vi "Client Close.vi"(8 "error in":errorcluster, 11 "connection ID":T1) -> (0 "error out":errorcluster)   [LabVIEW 2010, in "NI_CCC.lvlib"]
doc: "Closes the connection with the server."
uses:
  NI_CCC.lvlib
  Connection ID.ctl
  <vilib>/NI/STM/TCP/TCP Connection Info.ctl
  <vilib>/NI/STM/SubVIs/MetaDataElement.ctl
  Tag Configuration.ctl
  <vilib>/NI/Current Value Table/Type Defs/Data Types.ctl
  Tag Direction.ctl
  FG Client Configurations Action.ctl
  <vilib>/NI/STM/TCP/TCP Write Options.ctl
  <vilib>/NI/Current Value Table/FGVs/Group Memory.vi
  <vilib>/NI/STM/NI STM.lvlib
  <vilib>/NI/Current Value Table/Current Value Table.lvlib
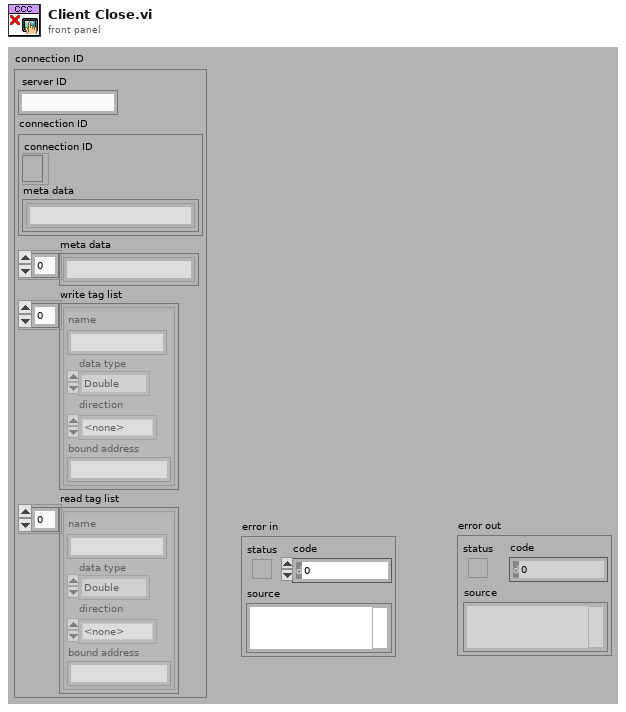
[diagram p1: front panel]
types:
  T1 = typedef "NI_CCC.lvlib/Connection ID.ctl" = cluster{"server ID":string, "connection ID":T2, "meta data":T3[], "write tag list":T4[], "read tag list":T4[]}
  T2 = typedef "NI STM.lvlib/TCP Connection Info.ctl" = cluster{"connection ID":refnum<k5>, "meta data":T3[]}
  T3 = typedef "NI STM.lvlib/MetaDataElement.ctl" = string
  T4 = typedef "NI_CCC.lvlib/Tag Configuration.ctl" = cluster{"name":string, "data type":T5, "direction":T6, "bound address":string}
  T5 = typedef "Current Value Table.lvlib/Data Types.ctl" = enum16{"Double", "Single", "I64", "I32", "I16", "I8", "U64", "U32", "U16", "U8", "String", "Boolean", "Array of U8", "Array of U16", "Array of U32", "Array of U64", "Array of I64", "Array of I32", "Array of I16", "Array of I8", "Array of Double", "Array of Single", "Array of Boolean", "Array of String"}
  T6 = typedef "NI_CCC.lvlib/Tag Direction.ctl" = enum32{"<none>", "Read", "Write"}
  T7 = typedef "NI_CCC.lvlib/FG Client Configurations Action.ctl" = enum16{"Check Read Config", "Check Write Config", "Mark Read Config", "Mark Write Config"}
  T8 = typedef "NI STM.lvlib/TCP Write Options.ctl" = cluster{"ignore timeout error":bool, "timeout ms (1000)":i32}
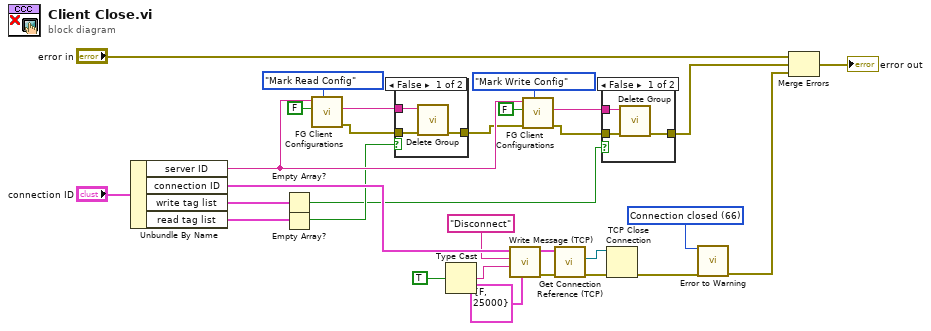
[diagram p0: block diagram]
diagram:
  w27 = 66 items=["No Error", "Argument Error", "Memory Full", "Out of Zone", "End of File", "File Already Open", "Generic File IO Error", "File Not Found", "File Permission Error", "Disk Full", "Duplicate Path", "Too Many Files Open", "Not Enabled", "Resource File Not Found", "Cannot Add Resource", "Resource Not Found", "Image Not Found", "Image Memory Error", "Pen Does Not Exist", "Config Bad Type", "Config Token Not Found", "Config Parse Error", "Config Memory Error", "Bad External Code Format", "Bad External Code Offset", "External Code Not Present", "Null Window", "Destroy Window Mixup", "Null Menu", "Print Aborted", "Bad Print Record", "Print Driver Error", "Windows Error During Print", "Memory Error During Print", "Print Dialog Error", "Generic Print Error", "Invalid Device Refnum", "Device Not Found", "Device Parameter Error", "Device Unit Error", "Can't Open Device", "Device Call Aborted", "Generic Error", "Cancelled By User", "Object ID Too Low", "Object ID Too High", "Object Not In Heap", "Unknown Heap", "Bad DefProc ID", "DefProc Not In Table", "Message Out Of Range", "Null Method", "Unknown Message", "Manager Call Not Supported", "Bad address", "Connection In progress", "Connection timed out", "Connection is already in progress", "Network attribute not supported", "Network error", "Address in use", "System out of memory", "Connection aborted", "Connection refused", "Connection is not connected", "Connection is already connected", "Connection closed", "Initialize error (interapplication manager)", "Bad occurrence", "Wait on unbound occurrence handler", "Occurrence queue overflow", "Bad path", "Semaphore not signaled", "Unrecognized type (interapplication manager)"] ("1st Error to Convert")
  n1 = Unbundle By Name("connection ID") -> ("server ID"=w16:string, "connection ID"=w29:T2, "write tag list"=w4:T4[], "read tag list"=w3:T4[])
  n2 = Empty Array?(array=w4) -> (empty?=w1:bool)
  n3 = Empty Array?(array=w3) -> (empty?=w2:bool)
  n4 = call "FG Client Configurations.vi"("action"=FG_Client_Configurations_Action."Mark Read Config", "mark configured? (T)"=FALSE, "server ID"=w16) -> ("error out"=w9:errorcluster, "group name"=w15:string)  [unwired: 6 in, 1 out]
  n5 = case shown="False" w2 {
    tunnel: w15 -> [w33 _]
    tunnel: w9 -> [w32 w34]
    tunnel: [w31 w34] -> w8
    frame False {
      n6 = call <vilib>:"Delete Group.vi"("error in (no error)"=w32, "Group"=w33) -> ("error out"=w31:errorcluster)  [unwired: 9 in]
    }
    frame True {
    }
  }
  n7 = Type Cast(x=TRUE ("Stop?")) -> (*(type *) &x=w25:string)  [unwired: 1 out]
  n8 = call <vilib>:"Write Message (TCP).vi"("options"=T8 {"ignore timeout error"=FALSE, "timeout ms (1000)"=25000} ("Options"), "data"=w25, "name"="Disconnect" ("Name"), "connection info in"=w29) -> ("error out"=w22:errorcluster, "connection info out"=w20:T2)  [unwired: 6 in]
  n9 = call "FG Client Configurations.vi"("action"=FG_Client_Configurations_Action."Mark Write Config", "error in"=w8, "mark configured? (T)"=FALSE, "server ID"=w16) -> ("error out"=w7:errorcluster, "group name"=w14:string)  [unwired: 5 in, 1 out]
  n10 = call <vilib>:"Get Connection Reference (TCP).vi"("error in"=w22, "connection info in"=w20) -> ("error out"=w21:errorcluster, "connection ID out"=w19:refnum<k5>)  [unwired: 7 in, 1 out]
  n11 = case shown="False" w1 {
    tunnel: w14 -> [w37 _]
    tunnel: w7 -> [w36 w38]
    tunnel: [w35 w38] -> w5
    frame False {
      n12 = call <vilib>:"Delete Group.vi"("error in (no error)"=w36, "Group"=w37) -> ("error out"=w35:errorcluster)  [unwired: 9 in]
    }
    frame True {
    }
  }
  n13 = TCP Close Connection(connection ID=w19, error in (no error)=w21) -> (error out=w26:errorcluster)  [unwired: 2 out]
  n14 = call <vilib>:"Error to Warning.vi"("1st Error to Convert"=w27, "error in"=w26) -> ("warning out"=w6:errorcluster)  [unwired: 3 in, 10 out]
  n15 = Merge Errors("error in", w5, w6) -> (→"error out":errorcluster)
